vi "ParseSysexMsgPinStateResponse.vi"(8 "error in":errorcluster, 10 "Sysex Message":u8[](array[numeric]) format="%x") -> (0 "error out":errorcluster, 1 "Pin State":u64, 2 "Pin Index":u8, 4 "Pin Mode":T1=enum."Extended.DHT")   [LabVIEW 2020]
doc: "Parse a message according to the Firmata Protocol Requirements. \n- https://github.com/firmata/protocol\n- https://github.com/firmata/protocol/blob/master/protocol.md"
uses:
  Controls/FirmataPinModes.ctl
  Controls/FirmataProtocolConstants.ctl
panel:
  out "IsValidSysex":bool
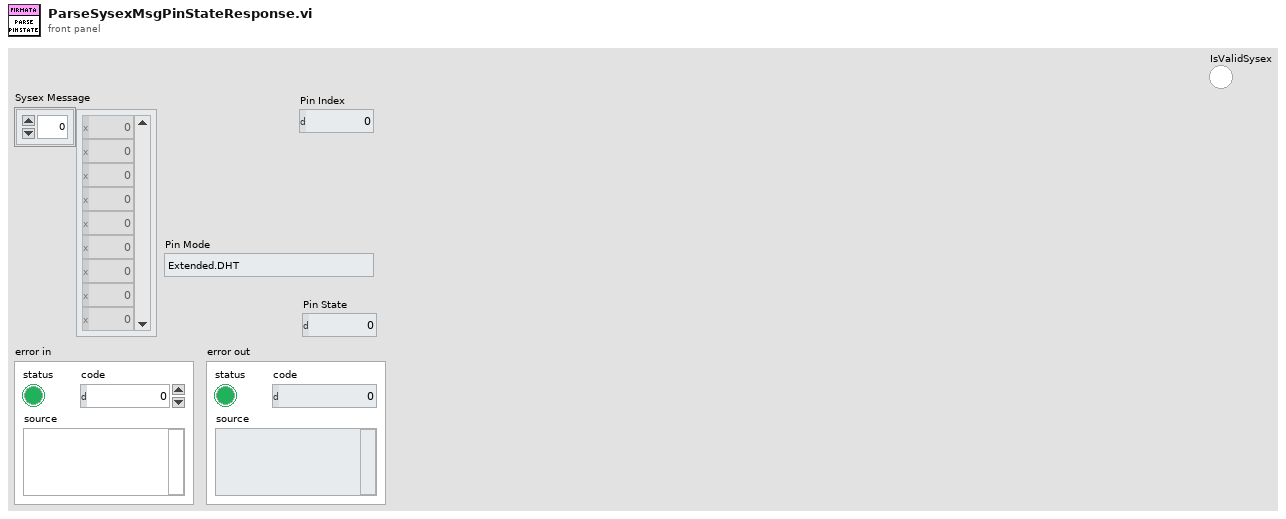
[diagram p1: front panel]
types:
  T1 = typedef "FirmataPinModes.ctl" = enum16{"DigitalInput", "DigitalOutput", "AnalogInput", "PWM", "Servo", "Shift", "I2C", "OneWire", "Stepper", "Encoder", "Serial", "InputPullup", "Extended.SPI", "Extended.Sonar", "Extended.Tone", "Extended.DHT"}
  T2 = typedef "FirmataProtocolConstants.ctl" = u16
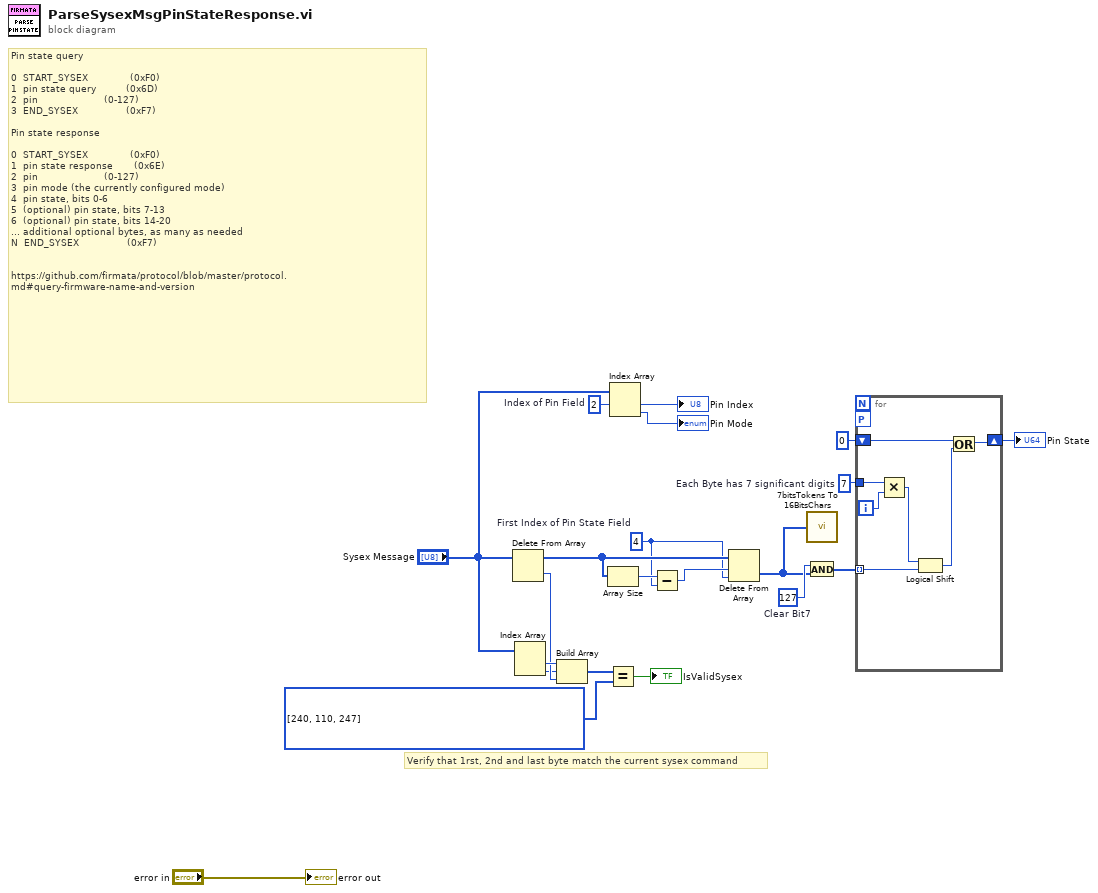
[diagram p0: block diagram]
diagram:
  w4 = T2[] [240, 110, 247] items=["ANALOG_IO_MESSAGE"=224, "DIGITAL_IO_MESSAGE"=144, "REPORT_ANALOG_PIN"=192, "REPORT_DIGITAL_PORT"=208, "START_SYSEX"=240, "END_SYSEX"=247, "SET_PIN_MODE"=244, "SET_DIGITAL_PIN_VALUE"=245, "PROTOCOL_VERSION"=249, "SYSTEM_RESET"=255, "SYSEX.EXTENDED_ID"=0, "SYSEX.RESERVED_USER_COMMANDs"=1, "SYSEX.ANALOG_MAPPING_QUERY"=105, "SYSEX.ANALOG_MAPPING_RESPONSE"=106, "SYSEX.CAPABILITY_QUERY"=107, "SYSEX.CAPABILITY_RESPONSE"=108, "SYSEX.PIN_STATE_QUERY"=109, "SYSEX.PIN_STATE_RESPONSE"=110, "SYSEX.REPORT_FIRMWARE"=121, "SYSEX.EXTENDED_ANALOG"=111, "SYSEX.STRING_DATA"=113, "SYSEX.REALTIME"=127, "SYSEX.NON_REALTIME"=126, "SYSEX.SAMPLING_INTERVAL"=122, "FEATURES.SYSEX.I2C_READ_WRITE"=118, "FEATURES.SYSEX.I2C_REPLY"=119, "FEATURES.SYSEX.I2C_CONFIG"=120]
  w6 = u8 7  # Each Byte has 7 significant digits
  w9 = u8 127  # Clear Bit7
  w10 = 4  # First Index of Pin State Field
  w13 = 2  # Index of Pin Field
  # "Verify that 1rst, 2nd and last byte match the current sysex command"
  # "Pin state query\n\n0  START_SYSEX              (0xF0)\n1  pin state query          (0x6D)\n2  pin                      (0-127)\n3  END_SYSEX                (0xF7)\n\nPin state response\n\n0  START_SYSEX              (0xF0)\n1  pin state response       (0x6E)\n2  pin                      (0-127)\n3  pin mode (the currently configured mode)\n4  pin state, bits 0-6\n5  (optional) pin state, bits 7-13\n6  (optional) pin state, bits 14-20\n... additional optional bytes, as many as needed\nN  END_SYSEX                (0xF7)\n\n\nhttps://github.com/firmata/protocol/blob/master/protocol.md#query-firmware-name-and-version"
  n1 = Delete From Array(array="Sysex Message") -> (deleted portion=w19:u8, array with subset deleted=w15:u8[])  [unwired: 2 in]
  n2 = Index Array(array="Sysex Message") -> (element #1=w20:u8, element #2=w18:u8)  [unwired: 2 in]
  n3 = Build Array(w20, w18, w19) -> (w17:u8[])
  n4 = Array Size(array=w15) -> (size(s)=w14:i32)
  n5 = Equal?(x=w17, y=w4) -> (x = y?=→"IsValidSysex":bool)
  n6 = Index Array(array="Sysex Message", index #1=w13) -> (element #1=→"Pin Index":u8, element #2=→"Pin Mode":u8)  [unwired: 1 in]
  n7 = Subtract(x=w14, y=w10) -> (x-y=w11:i32)
  n8 = Delete From Array(array=w15, length=w11, index=w10) -> (deleted portion=w2:u8[])  [unwired: 1 out]
  n9 = call "7bitsTokens To 16BitsChars.vi"("Bytes In"=w2) -> ()  [unwired: 1 out]
  n10 = And(x=w9, y=w2) -> (x .and. y?=w8:u8[])
  n11 = for {
    tunnel: w8 -> [w26] mode=indexing
    shift-right: [w27] -> w1
    shift-left: u64 0 -> [w28]
    tunnel: w6 -> [w24]
    workers-P: _ -> [_]
    i -> [w23]
    n12 = Multiply(x=w24, y=w23) -> (x*y=w22:i32)
    n13 = Logical Shift(y=w22, x=w26) -> (x << y=w25:u8)
    n14 = Or(x=w28, y=w25) -> (x .or. y?=w27:u64)
  }
  "Pin State" <- w1
  "error out" <- "error in"
